vi "EPNH354_LabMotorDriver_Sub-VI.vi"(0 "LINX Resource in":T1, 1 "Array":i32[](array[numeric]), 2 "Step Size in":dbl, 5 "Run Clockwise in":bool, 7 "Rotation Range in":dbl, 9 "Run Continuous in":bool, 11 "error in (no error)":errorcluster, 12 "Wait [ms] in":i64, 13 "stop in":bool) -> (4 "LINX Resource out":T1, 15 "error out":errorcluster)   [LabVIEW 2020]
uses:
  <vilib>/MakerHub/LINX/Private/Type Defs/LINX Ref.ctl
  <vilib>/MakerHub/LINX/Private/Type Defs/Platform.ctl
  <vilib>/MakerHub/LINX/Private/Type Defs/Interface.ctl
  <vilib>/MakerHub/LINX/Private/Device/Type Defs/LINX Device Config.ctl
  <vilib>/MakerHub/LINX/Private/Device/Type Defs/TCP Config.ctl
  <vilib>/MakerHub/LINX/Private/Device/Type Defs/Channels.ctl
  <vilib>/MakerHub/LINX/Public/Peripherals/Digital/Digital Write N Chans.vi
  <vilib>/MakerHub/LINX/Private/Local IO/LinxDigitalWrite.vi
  <vilib>/MakerHub/LINX/Public/Utilities/Check Channel.vi
  <vilib>/MakerHub/LINX/Private/Utilties/Generate Error.vi
  <vilib>/MakerHub/LINX/LMH-LINX.lvlib
  <vilib>/MakerHub/LINX/Private/Device/Device.lvlib
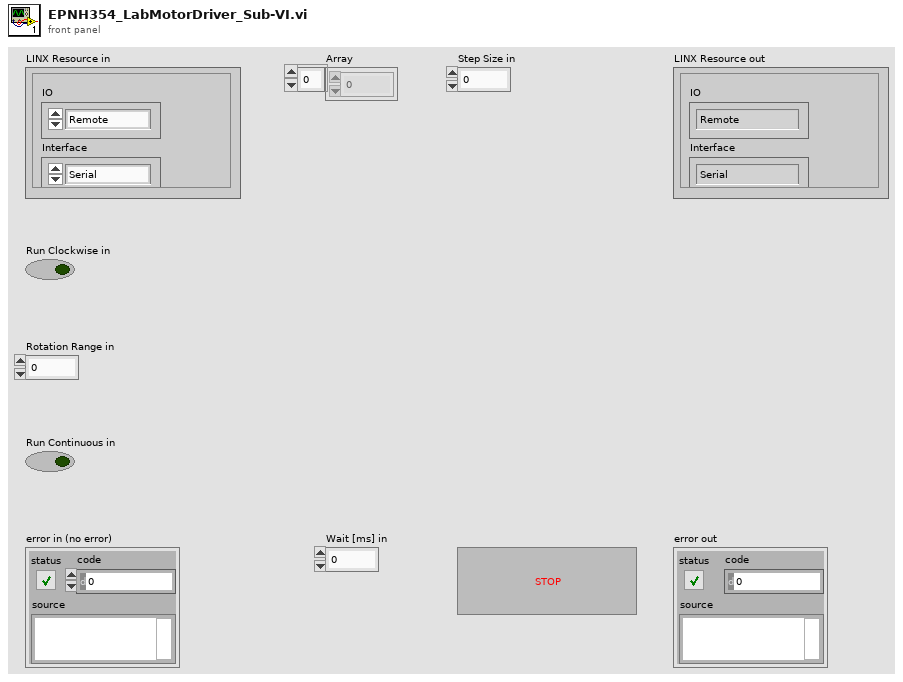
[diagram p1: front panel]
types:
  T1 = typedef "LMH-LINX.lvlib/LINX Ref.ctl" = cluster{"IO":T2, "Interface":T3, "LINX Device Config":T4}
  T2 = typedef "LMH-LINX.lvlib/Platform.ctl" = enum16{"Remote", "Local"}
  T3 = typedef "LMH-LINX.lvlib/Interface.ctl" = enum16{"Serial", "TCP"}
  T4 = typedef "LMH-LINX.lvlib/Device.lvlib/LINX Device Config.ctl" = cluster{"Interface":T3, "COM Port":refnum<visa-resource-name>, "TCP Configuration":T5, "Device Family":u8, "Device ID":u8, "Device Name":string, "TCP Ref":refnum<k5>, "Channels":T6}
  T5 = typedef "LMH-LINX.lvlib/Device.lvlib/TCP Config.ctl" = cluster{"IP Address":string, "Port":u16}
  T6 = typedef "LMH-LINX.lvlib/Channels.ctl" = cluster{"DI":u8[], "DO":u8[], "AI":u8[], "AO":u8[], "PWM":u8[], "QE":u8[], "UART":u8[], "I2C 2":u8[], "SPI":u8[], "CAN":u8[], "Servo":u8[], "AI Ref (V)":dbl, "AI Resolution (Bits)":u8, "AO Ref (V)":dbl, "AO Resolution (Bits)":u8}
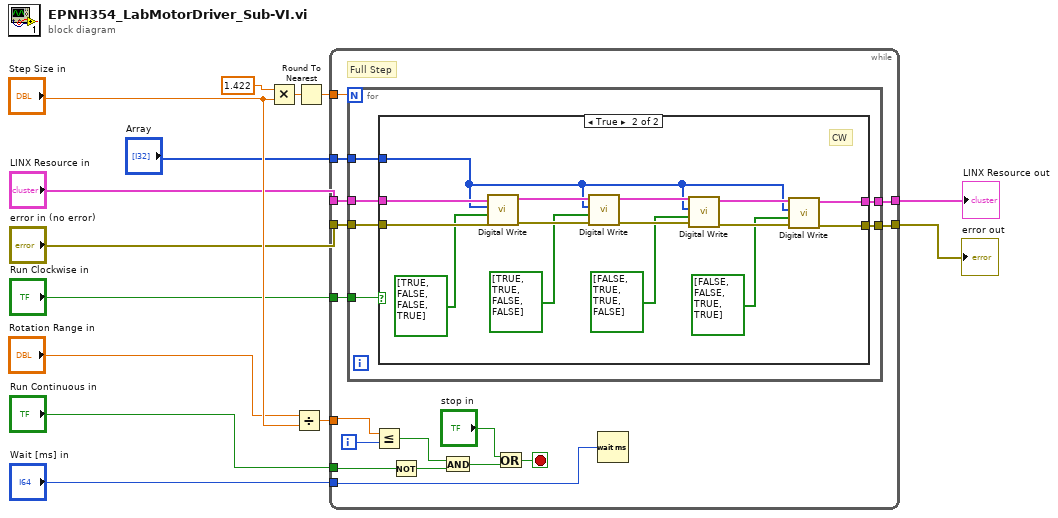
[diagram p0: block diagram]
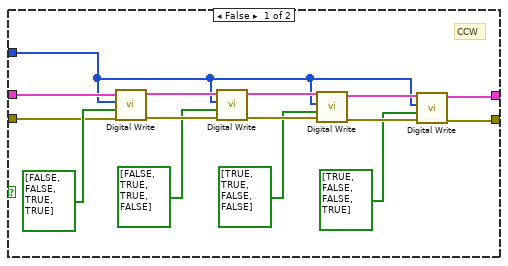
[diagram p2: hidden frame]
diagram:
  n1 = Multiply(x=1.422 ("y"), y="Step Size in") -> (x*y=w7:dbl)
  n2 = Divide(x="Rotation Range in", y="Step Size in") -> (x/y=w13:dbl)
  n3 = Round To Nearest(number=w7) -> (nearest integer value=w8:dbl)
  n4 = while {
    tunnel: "error in (no error)" -> [w28]
    tunnel: "LINX Resource in" -> [w30]
    tunnel: [w29] -> w3
    tunnel: [w27] -> w4
    tunnel: "Array" -> [w26]
    tunnel: w8 -> [w22]
    tunnel: "Run Continuous in" -> [w18]
    tunnel: "Run Clockwise in" -> [w23]
    tunnel: w13 -> [w20]
    tunnel: "Wait [ms] in" -> [w15]
    i -> [w19]
    stop <- w25 stop-if-true
    # "Full Step"
    n5 = for {
      N: w22 -> [_]
      tunnel: w30 -> [w36]
      tunnel: [w35] -> w29
      tunnel: w28 -> [w34]
      tunnel: [w33] -> w27
      tunnel: w26 -> [w32]
      tunnel: w23 -> [w31]
      n6 = case shown="True" w31 {
        tunnel: w36 -> [w41 w60]
        tunnel: [w39 w59] -> w35
        tunnel: w34 -> [w40 w58]
        tunnel: [w38 w57] -> w33
        tunnel: w32 -> [w37 w52]
        frame False {
          # "CCW"
          n7 = call-poly <vilib>:"Digital Write.vi"("Error In"=w40, "Values"=bool[] [FALSE, FALSE, TRUE, TRUE], "DO Channels"=w37, "LINX Resource"=w41) -> ("Error Out"=w48:errorcluster, "LINX Resource"=w51:T1)  [unwired: 6 in]
          n8 = call-poly <vilib>:"Digital Write.vi"("Error In"=w48, "Values"=bool[] [FALSE, TRUE, TRUE, FALSE], "DO Channels"=w37, "LINX Resource"=w51) -> ("Error Out"=w47:errorcluster, "LINX Resource"=w50:T1)  [unwired: 6 in]
          n9 = call-poly <vilib>:"Digital Write.vi"("Error In"=w47, "Values"=bool[] [TRUE, TRUE, FALSE, FALSE], "DO Channels"=w37, "LINX Resource"=w50) -> ("Error Out"=w46:errorcluster, "LINX Resource"=w49:T1)  [unwired: 6 in]
          n10 = call-poly <vilib>:"Digital Write.vi"("Error In"=w46, "Values"=bool[] [TRUE, FALSE, FALSE, TRUE], "DO Channels"=w37, "LINX Resource"=w49) -> ("Error Out"=w38:errorcluster, "LINX Resource"=w39:T1)  [unwired: 6 in]
        }
        frame True {
          # "CW"
          n11 = call-poly <vilib>:"Digital Write.vi"("Error In"=w58, "Values"=bool[] [TRUE, FALSE, FALSE, TRUE], "DO Channels"=w52, "LINX Resource"=w60) -> ("Error Out"=w63:errorcluster, "LINX Resource"=w66:T1)  [unwired: 6 in]
          n12 = call-poly <vilib>:"Digital Write.vi"("Error In"=w63, "Values"=bool[] [TRUE, TRUE, FALSE, FALSE], "DO Channels"=w52, "LINX Resource"=w66) -> ("Error Out"=w62:errorcluster, "LINX Resource"=w65:T1)  [unwired: 6 in]
          n13 = call-poly <vilib>:"Digital Write.vi"("Error In"=w62, "Values"=bool[] [FALSE, TRUE, TRUE, FALSE], "DO Channels"=w52, "LINX Resource"=w65) -> ("Error Out"=w61:errorcluster, "LINX Resource"=w64:T1)  [unwired: 6 in]
          n14 = call-poly <vilib>:"Digital Write.vi"("Error In"=w61, "Values"=bool[] [FALSE, FALSE, TRUE, TRUE], "DO Channels"=w52, "LINX Resource"=w64) -> ("Error Out"=w57:errorcluster, "LINX Resource"=w59:T1)  [unwired: 6 in]
        }
      }
    }
    n15 = Less Or Equal?(x=w20, y=w19) -> (x <= y?=w21:bool)
    n16 = Not(x=w18) -> (.not. x?=w17:bool)
    n17 = And(x=w21, y=w17) -> (x .and. y?=w16:bool)
    n18 = Or(x="stop in", y=w16) -> (x .or. y?=w25:bool)
    n19 = Wait (ms)(milliseconds to wait=w15) -> ()  [unwired: 1 out]
  }
  "error out" <- w4
  "LINX Resource out" <- w3
